vi "User_Metadata.vi"() -> ()   [LabVIEW 2010]
uses:
  ADAM Controls/Channel_names.ctl
  ADAM Controls/Module_type_ADAM.ctl
  ADAM Controls/Channel_State.ctl
  ADAM Controls/Calib_type_ADAM.ctl
  Anemometry/Anemometry Sub Vis/Controls/Preference_Mode.ctl
  ADAM Controls/Update_scan_value.ctl
  Anemometry/Anemometry Sub Vis/Globals/Preference_global.vi
  Anemometry/Anemometry Sub Vis/Globals/Constants_global.vi
  Anemometry/Anemometry Sub Vis/Globals/Meas_global.vi
  Anemometry/Anemometry Sub Vis/Globals/Trav_pos_global.vi
panel:
  in  "Edit Preference Panel":bool
  out "Rig Name":string="EnFlo Tunnel"
  in  "Edit Email Addresses":bool
  out "Email Addresses":string[](array[string])
  in  "Value 10":string
  in  "Value 9":string
  in  "Value 8":string
  in  "Value 7":string
  in  "Value 6":string
  in  "Menu 10":u16(ring) items=["Edit Strings", "20mm Cubes"]
  out "Channel Name 10":string
  in  "Menu 9":u16(ring) items=["Edit Strings", "None", "Ramp 29 x 390mm", "Ramp 9 x 175mm", "Rounded nose 18.2 x 55mm", "Rounded nose 9 x 150mm"]
  out "Channel Name 9":string
  in  "Menu 8":u16(ring) items=["Edit Strings", "20mm Cubes"]
  out "Channel Name 8":string
  in  "Menu 7":u16(ring) items=["Edit Strings", "0", "115", "65"]
  out "Channel Name 7":string
  in  "Menu 6":u16(ring) items=["Edit Strings", "0", "1", "16"]
  out "Channel Name 6":string
  out "Clear remaining channels":bool
  in  "Value 5":string
  in  "Menu 5":u16(ring) items=["Edit Strings", "0", "25", "6.25"]
  out "Channel Name 5":string
  in  "Value 4":string
  in  "Menu 4":u16(ring) items=["Edit Strings", "20 x 20mm", "40 x 40mm", "80 x 80mm", "None"]
  out "Channel Name 4":string
  in  "Value 3":string
  in  "Menu 3":u16(ring) items=["Edit Strings", "0", "10", "20", "Normal distribution with average = 10mm"]
  out "Channel Name 3":string
  in  "Value 2":string
  in  "Menu 2":u16(ring) items=["Edit Strings", "None", "Random blocks", "Uniform cube"]
  out "Channel Name 2":string
  in  "Modify User Channels":bool
  out "Channel No":i32
  out "First Loop":bool
  out "Index":i32
  in  "Value 1":string
  in  "Menu 1":u16(ring) items=["Edit Strings", "Aligned", "None", "Staggered"]
  out "Channel Name 1":string
  in  "stop":bool
  in  "OK":bool
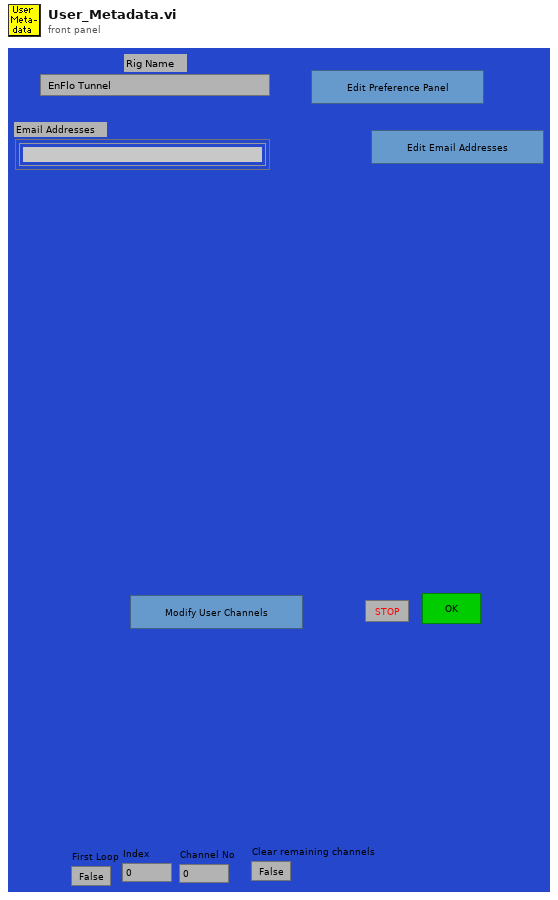
[diagram p1: front panel]
types:
  T1 = typedef "Channel_names.ctl" = enum16{"Active Only", "Active + Off", "All Channels"}
  T2 = typedef "Calib_type_ADAM.ctl" = enum16{"Raw", "Bx + A", "Cx^2 + Bx + A", "Dx^3 + Cx^2 + Bx + A", "In Band", "Hi-Tec Q", "Hi-Tec M_dot", "Text"}
  T3 = typedef "Preference_Mode.ctl" = enum16{"Load Preferences from file", "Save Preferences to file", "Load, Edit then Save"}
  T4 = typedef "Channel_State.ctl" = enum16{"On", "Off", "Always On", "Always Off"}
  T5 = typedef "Module_type_ADAM.ctl" = enum16{"4011", "4012", "4013", "4014", "4016", "4017", "4018", "4021", "4050", "4052", "4053", "4060", "4080", "5000", "5017", "5018", "5024", "5051", "5056", "5060", "6060", "Tracker", "WEST", "GILL", "JEM", "VICI", "Vaisala", "DRUCK", "Run VI Named:", "IR2100", "PPT", "Comparator", "VIRTUAL", "Hold Value", "Read A", "Read Ch", "Coded", "Client Info", "Web Client", "X10", "Test"}
  T6 = typedef "Ch_description_ADAM.ctl" = cluster{"Ch Name":string, "Type":T5, "Function":T7, "Ch State":T4, "Calibration type":T2, "A":dbl, "B":dbl, "C":dbl, "D":dbl, "Comments":string, "Address":T8, "String":string, "Duty":u16}
  T7 = typedef "Function_ADAM.ctl" = enum16{"Analogue Input", "Digital Input", "Event counter", "Event rate", "Analogue Output", "Digital Output", "Relay Output"}
  T8 = typedef "Address.ctl" = cluster{"Main":i32, "Ch.":i32, "Sub":i32, "Port Name":string}
  T9 = typedef "Update_scan_value.ctl" = cluster{"Channel Name":string, "New Value":dbl}
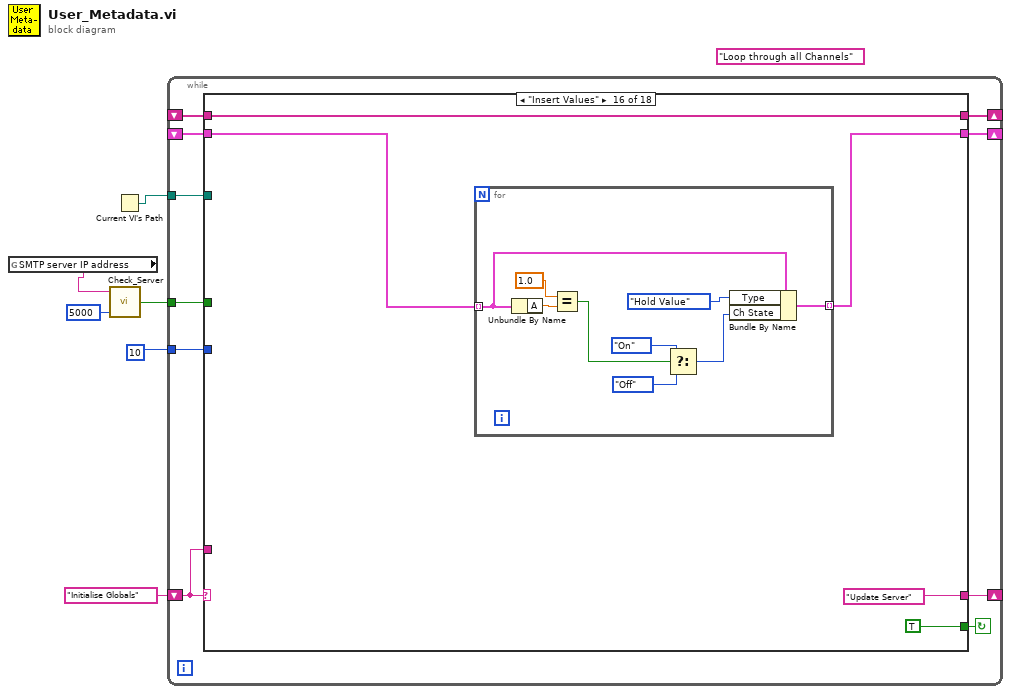
[diagram p0: block diagram]
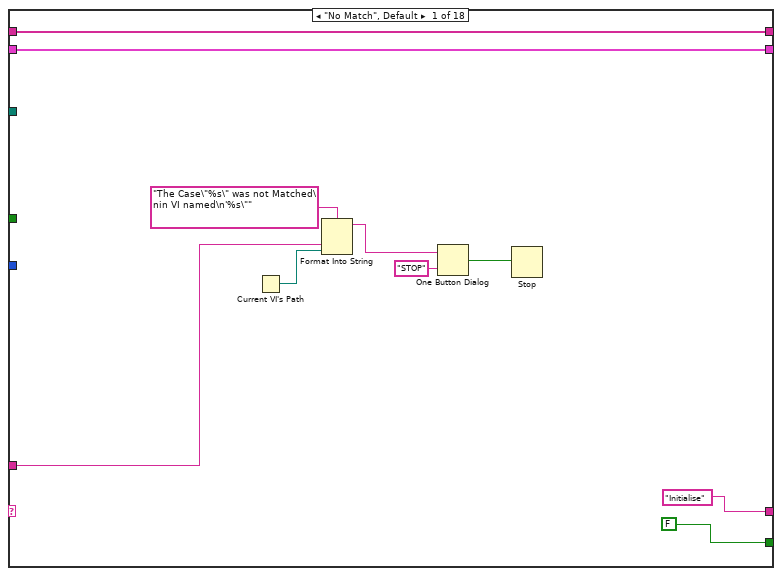
[diagram p2: hidden frame]
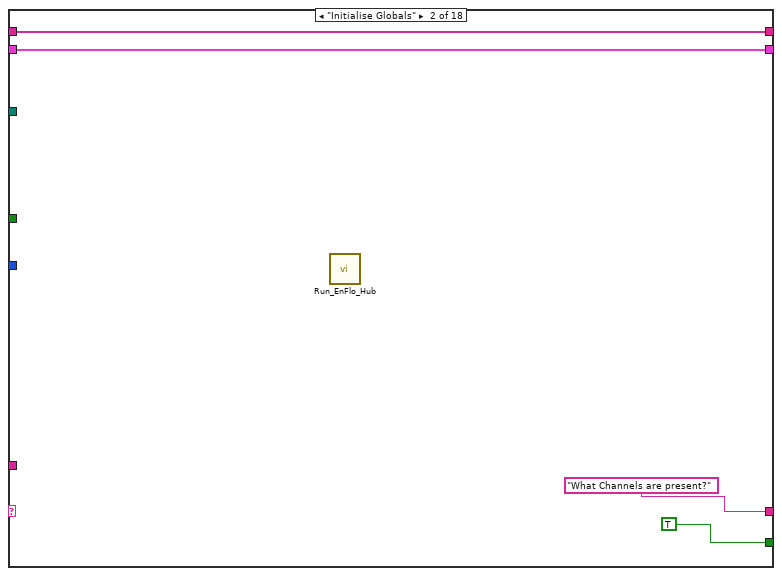
[diagram p3: hidden frame]
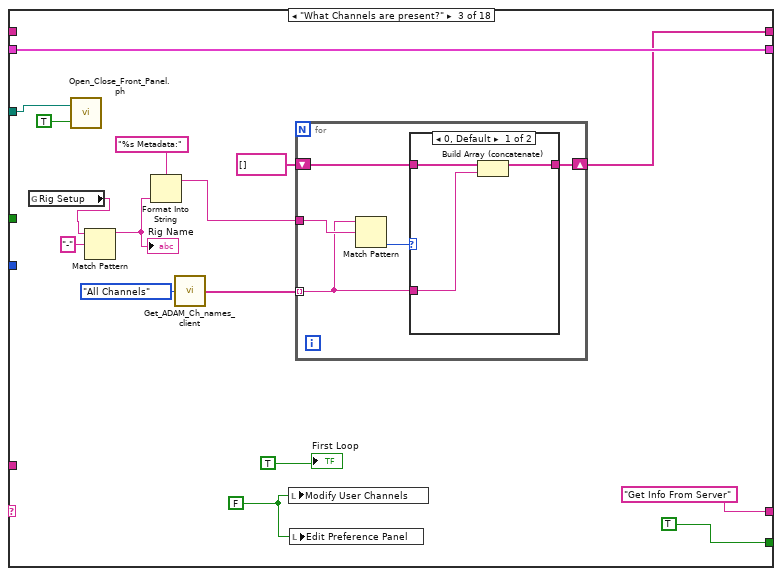
[diagram p4: hidden frame]
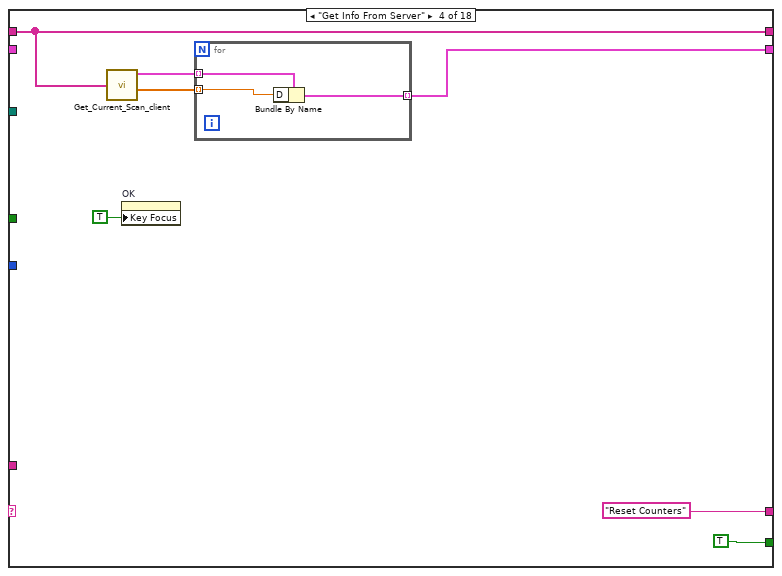
[diagram p6: hidden frame]
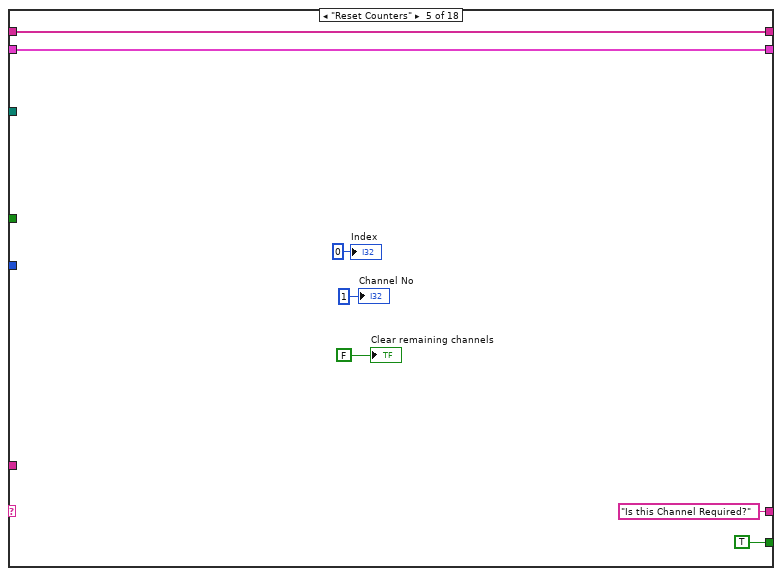
[diagram p7: hidden frame]
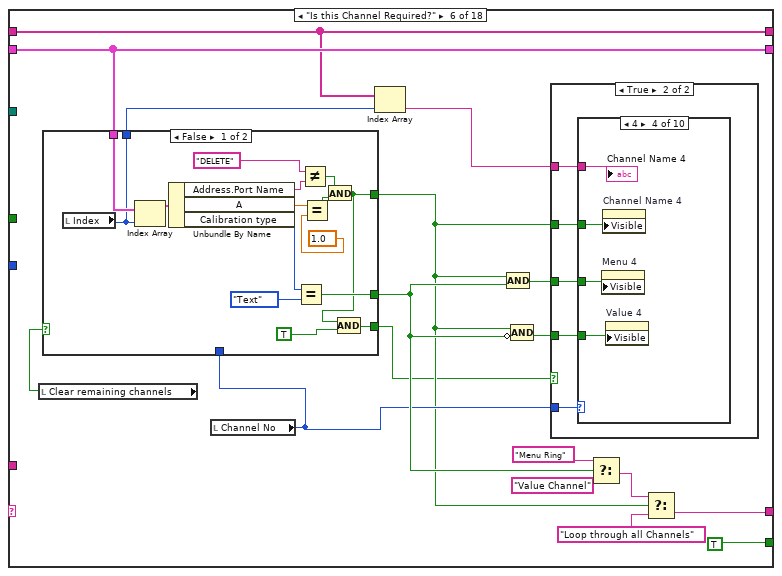
[diagram p8: hidden frame]
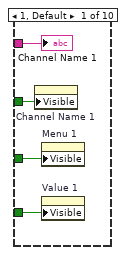
[diagram p10: hidden frame]
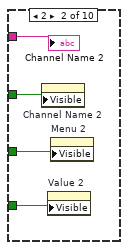
[diagram p11: hidden frame]
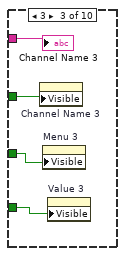
[diagram p12: hidden frame]
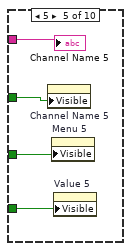
[diagram p13: hidden frame]
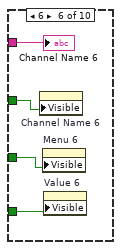
[diagram p14: hidden frame]
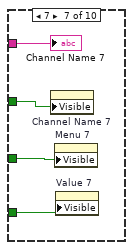
[diagram p15: hidden frame]
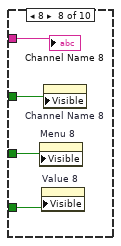
[diagram p16: hidden frame]
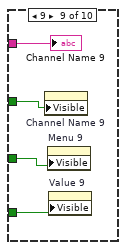
[diagram p17: hidden frame]
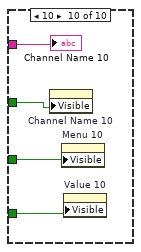
[diagram p18: hidden frame]
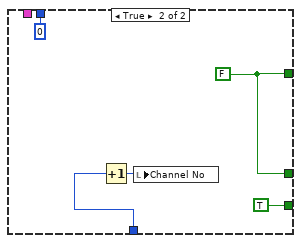
[diagram p19: hidden frame]
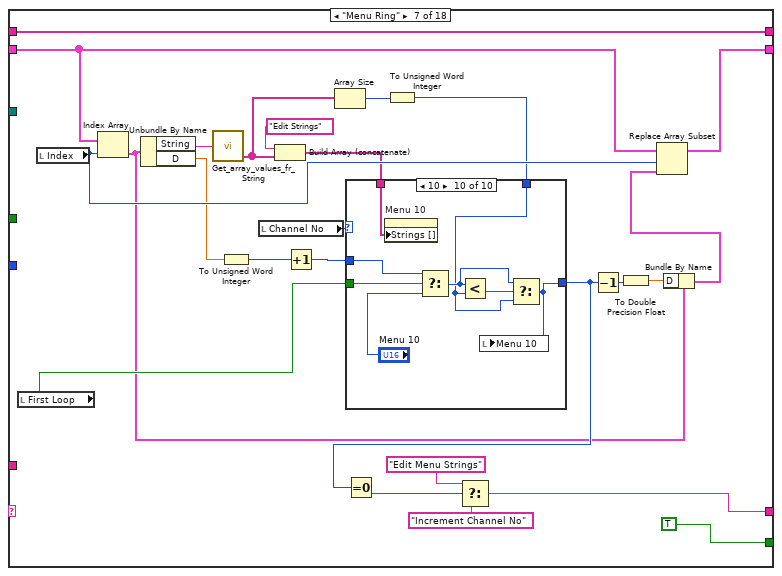
[diagram p20: hidden frame]
diagram:
  (unwired) "Loop through all Channels"
  n1 = global read "Preference_global.vi" "SMTP server IP address"() -> (w2:string)
  n2 = call "Check_Server.vi"("timeout ms (60000)"=5000, "address"=w2) -> ("OK"=w1:bool)  [unwired: 3 out]
  n3 = Current VI's Path() -> (path=w4:path)
  n4 = while {
    tunnel: 10 -> [w9]
    shift-left: _ -> [w12]
    shift-right: [w11] -> _
    shift-left: _ -> [w13]
    shift-right: [w14] -> _
    shift-left: "Initialise Globals" -> [w15]
    shift-right: [w10] -> _
    tunnel: w4 -> [w8]
    tunnel: w1 -> [w7]
    stop <- w16 continue-if-true
    n5 = case shown="\"Insert Values\"" w15 {
      tunnel: [FALSE TRUE TRUE TRUE TRUE ("T button?") TRUE TRUE TRUE TRUE TRUE TRUE TRUE TRUE TRUE ("T button?") TRUE ("T button?") TRUE ("T button?") TRUE ("T button?") FALSE ("T button?")] -> w16
      tunnel: ["Initialise" "What Channels are present?" "Get Info From Server" "Reset Counters" "Is this Channel Required?" w84 w166 "Increment Channel No" "Increment Channel No" "Loop through all Channels" w347 "What Channels are present?" "Reset Counters" w396 "Insert Values" "Update Server" w439 "End"] -> w10
      tunnel: w15 -> [w21 _ _ _ _ _ _ _ _ _ _ _ _ _ _ _ _ _]
      tunnel: [w18 w28 w44 w57 w69 w88 w158 w269 w287 w345 w358 w379 w384 w406 w419 w427 w440 w487] -> w14
      tunnel: w13 -> [w18 w28 w44 _ w69 w88 w159 w268 w288 w345 w358 w379 w385 w406 w419 w425 w440 w487]
      tunnel: w12 -> [w17 w27 _ w60 w70 w78 w178 w273 w298 w344 w363 w380 _ w399 w417 w426 w441 w488]
      tunnel: [w17 w27 w40 w60 w70 w78 w178 w273 w298 w344 w363 w380 w383 w399 w417 w426 w441 w488] -> w11
      tunnel: w9 -> [_ _ _ _ _ _ _ _ _ _ w353 _ _ _ _ _ _ _]
      tunnel: w8 -> [_ _ w35 _ _ _ _ _ _ _ _ _ _ _ _ _ _ w485]
      tunnel: w7 -> [_ _ _ _ _ _ _ _ _ _ _ _ _ _ w412 _ _ _]
      frame "No Match", Default {
        n6 = Current VI's Path() -> (path=w20:path)
        n7 = Format Into String(format string="The Case\"%s\" was not Matched\nin VI named\n'%s\"" ("Format String"), w21, w20) -> (resulting string=w24:string)  [unwired: 2 in, 1 out]
        n8 = One Button Dialog(message=w24, button name ("OK")="STOP") -> (true=w22:bool)
        n9 = Stop(stop? (T)=w22) -> ()
      }
      frame "Initialise Globals" {
        n10 = call "Run_EnFlo_Hub.vi"() -> ()  [unwired: 8 out]
      }
      frame "What Channels are present?" {
        w34 = FALSE ("Add a New Channel")
        n11 = global read "Preference_global.vi" "Rig Setup"() -> (w32:string)
        n12 = call "Open_Close_Front_Panel.ph.vi"("Front Panel Window:Open"=TRUE, "VI path"=w35) -> ()  [unwired: 2 out]
        n13 = Match Pattern(string=w32, regular expression="-") -> (before substring=w31:string)  [unwired: 4 out]
        "Rig Name" <- w31
        n14 = Format Into String(format string="%s Metadata:" ("Format String"), w31) -> (resulting string=w37:string)  [unwired: 2 in, 1 out]
        n15 = call "Get_ADAM_Ch_names_client.vi"("Channel names set"=Channel_names."All Channels") -> ("Ch names"=w42:string[])
        n16 = local write "Modify User Channels"(w34) -> ()
        n17 = local write "Edit Preference Panel"(w34) -> ()
        n18 = for {
          tunnel: w37 -> [w51]
          tunnel: w42 -> [w49] mode=indexing
          shift-right: [w47] -> w40
          shift-left: string[] [] -> [w48]
          n19 = Match Pattern(string=w49, regular expression=w51) -> (offset past match=w50:i32)  [unwired: 4 out]
          n20 = case shown="0, Default" w50 {
            tunnel: w49 -> [w54 _]
            tunnel: w48 -> [w53 w55]
            tunnel: [w52 w55] -> w47
            frame 0, Default {
              n21 = Build Array (concatenate)(w53, w54) -> (w52:string[])
            }
            frame -1 {
            }
          }
        }
        "First Loop" <- TRUE ("First Loop")
      }
      frame "Get Info From Server" {
        n22 = call "Get_Current_Scan_client.vi"("ADAM Ch Names"=w60) -> ("Ch Description Array"=w59:T6[], "Numerical Values"=w58:dbl[])  [unwired: 2 out]
        n23 = property on="OK" class="Bool"("Key Focus"=TRUE) -> ()  [unwired: 2 in, 2 out]
        n24 = for {
          tunnel: w59 -> [w65] mode=indexing
          tunnel: w58 -> [w64] mode=indexing
          tunnel: [w63] -> w57 mode=indexing
          n25 = Bundle By Name(cluster=w65, "D"=w64) -> (w63:T6)
        }
      }
      frame "Reset Counters" {
        "Index" <- 0 ("Index")
        "Channel No" <- 1 ("Channel No")
        "Clear remaining channels" <- FALSE ("Clear remaining channels")
      }
      frame "Is this Channel Required?" {
        n26 = local read "Clear remaining channels"() -> (w76:bool)
        n27 = local read "Channel No"() -> (w75:i32)
        n28 = case shown="False" w76 {
          tunnel: w88 -> [w149 _]
          tunnel: [w135 w154] -> w74
          tunnel: [w145 w154] -> w83
          tunnel: [w144 0 ("Index")] -> w79
          tunnel: w75 -> [_ w151]
          tunnel: [w142 TRUE] -> w73
          frame False {
            n29 = local read "Index"() -> (w144:i32)
            n30 = Index Array(array=w149, index=w144) -> (element=w148:T6)
            n31 = Unbundle By Name(w148) -> ("Address.Port Name"=w139:string, "A"=w141:dbl, "Calibration type"=w146:T2)
            n32 = Equal?(x=w146, y=Calib_type_ADAM."Text" ("Calibration Type")) -> (x = y?=w145:bool)
            n33 = Not Equal?(x="DELETE", y=w139) -> (x != y?=w136:bool)
            n34 = Equal?(x=w141, y=1.0 ("x")) -> (x = y?=w137:bool)
            n35 = And(x=w136, y=w137) -> (x .and. y?=w135:bool)
            n36 = Compound Arithmetic op=AND(w135, TRUE ("Input")) -> (w142:bool)
          }
          frame True {
            w154 = FALSE
            n37 = Increment(x=w151) -> (x+1=w152:i32)
            n38 = local write "Channel No"(w152) -> ()
          }
        }
        n39 = Index Array(array=w78, index=w79) -> (element=w77:string)
        n40 = Compound Arithmetic op=AND(w74, w83) -> (w86:bool)
        n41 = Compound Arithmetic op=AND(w74, invert w83) -> (w87:bool)
        n42 = case shown="True" w73 {
          tunnel: w87 -> [_ w94]
          tunnel: w86 -> [_ w93]
          tunnel: w74 -> [_ w92]
          tunnel: w77 -> [_ w91]
          tunnel: w75 -> [_ w90]
          frame False {
          }
          frame True {
            n43 = case shown="4" w90 {
              tunnel: w92 -> [w96 w100 w104 w108 w112 w117 w121 w125 w129 w133]
              tunnel: w94 -> [w98 w102 w106 w110 w114 w115 w119 w123 w127 w131]
              tunnel: w93 -> [w97 w101 w105 w109 w113 w116 w120 w124 w128 w134]
              tunnel: w91 -> [w95 w99 w103 w107 w111 w118 w122 w126 w130 w132]
              frame 1, Default {
                n44 = property on="Channel Name 1" class="Str"("Visible"=w96) -> ()  [unwired: 2 in, 2 out]
                n45 = property on="Menu 1" class="Ring (strict)"("Visible"=w97) -> ()  [unwired: 2 in, 2 out]
                n46 = property on="Value 1" class="Str"("Visible"=w98) -> ()  [unwired: 2 in, 2 out]
                "Channel Name 1" <- w95
              }
              frame 2 {
                n47 = property on="Channel Name 2" class="Str"("Visible"=w100) -> ()  [unwired: 2 in, 2 out]
                n48 = property on="Value 2" class="Str"("Visible"=w102) -> ()  [unwired: 2 in, 2 out]
                n49 = property on="Menu 2" class="Ring (strict)"("Visible"=w101) -> ()  [unwired: 2 in, 2 out]
                "Channel Name 2" <- w99
              }
              frame 3 {
                n50 = property on="Channel Name 3" class="Str"("Visible"=w104) -> ()  [unwired: 2 in, 2 out]
                n51 = property on="Menu 3" class="Ring (strict)"("Visible"=w105) -> ()  [unwired: 2 in, 2 out]
                n52 = property on="Value 3" class="Str"("Visible"=w106) -> ()  [unwired: 2 in, 2 out]
                "Channel Name 3" <- w103
              }
              frame 4 {
                n53 = property on="Menu 4" class="Ring (strict)"("Visible"=w109) -> ()  [unwired: 2 in, 2 out]
                n54 = property on="Channel Name 4" class="Str"("Visible"=w108) -> ()  [unwired: 2 in, 2 out]
                n55 = property on="Value 4" class="Str"("Visible"=w110) -> ()  [unwired: 2 in, 2 out]
                "Channel Name 4" <- w107
              }
              frame 5 {
                n56 = property on="Channel Name 5" class="Str"("Visible"=w112) -> ()  [unwired: 2 in, 2 out]
                n57 = property on="Menu 5" class="Ring (strict)"("Visible"=w113) -> ()  [unwired: 2 in, 2 out]
                n58 = property on="Value 5" class="Str"("Visible"=w114) -> ()  [unwired: 2 in, 2 out]
                "Channel Name 5" <- w111
              }
              frame 6 {
                n59 = property on="Channel Name 6" class="Str"("Visible"=w117) -> ()  [unwired: 2 in, 2 out]
                n60 = property on="Menu 6" class="Ring (strict)"("Visible"=w116) -> ()  [unwired: 2 in, 2 out]
                n61 = property on="Value 6" class="Str"("Visible"=w115) -> ()  [unwired: 2 in, 2 out]
                "Channel Name 6" <- w118
              }
              frame 7 {
                n62 = property on="Channel Name 7" class="Str"("Visible"=w121) -> ()  [unwired: 2 in, 2 out]
                n63 = property on="Menu 7" class="Ring (strict)"("Visible"=w120) -> ()  [unwired: 2 in, 2 out]
                n64 = property on="Value 7" class="Str"("Visible"=w119) -> ()  [unwired: 2 in, 2 out]
                "Channel Name 7" <- w122
              }
              frame 8 {
                n65 = property on="Menu 8" class="Ring (strict)"("Visible"=w124) -> ()  [unwired: 2 in, 2 out]
                n66 = property on="Value 8" class="Str"("Visible"=w123) -> ()  [unwired: 2 in, 2 out]
                n67 = property on="Channel Name 8" class="Str"("Visible"=w125) -> ()  [unwired: 2 in, 2 out]
                "Channel Name 8" <- w126
              }
              frame 9 {
                n68 = property on="Channel Name 9" class="Str"("Visible"=w129) -> ()  [unwired: 2 in, 2 out]
                n69 = property on="Menu 9" class="Ring (strict)"("Visible"=w128) -> ()  [unwired: 2 in, 2 out]
                n70 = property on="Value 9" class="Str"("Visible"=w127) -> ()  [unwired: 2 in, 2 out]
                "Channel Name 9" <- w130
              }
              frame 10 {
                n71 = property on="Channel Name 10" class="Str"("Visible"=w133) -> ()  [unwired: 2 in, 2 out]
                n72 = property on="Menu 10" class="Ring (strict)"("Visible"=w134) -> ()  [unwired: 2 in, 2 out]
                n73 = property on="Value 10" class="Str"("Visible"=w131) -> ()  [unwired: 2 in, 2 out]
                "Channel Name 10" <- w132
              }
            }
          }
        }
        n74 = Select(t="Menu Ring", s=w83, f="Value Channel") -> (s? t:f=w81:string)
        n75 = Select(t=w81, s=w74, f="Loop through all Channels") -> (s? t:f=w84:string)
      }
      frame "Menu Ring" {
        n76 = local read "First Loop"() -> (w176:bool)
        n77 = local read "Index"() -> (w171:i32)
        n78 = Index Array(array=w159, index=w171) -> (element=w156:T6)
        n79 = Unbundle By Name(w156) -> ("String"=w177:string, "D"=w160:dbl)
        n80 = call "Get_array_values_fr_String.vi"("String Value"=w177) -> ("String array"=w164:string[])  [unwired: 1 out]
        n81 = To Unsigned Word Integer(number=w160) -> (unsigned 16bit integer=w175:u16)
        n82 = local read "Channel No"() -> (w170:i32)
        n83 = Build Array (concatenate)("Edit Strings", w164) -> (w165:string[])
        n84 = Increment(x=w175) -> (x+1=w173:u16)
        n85 = Array Size(array=w164) -> (size(s)=w163:i32)
        n86 = To Unsigned Word Integer(number=w163) -> (unsigned 16bit integer=w162:u16)
        n87 = case shown="10" w170 {
          tunnel: w176 -> [w186 w195 w203 w211 w219 w227 w235 w243 w251 w259]
          tunnel: w173 -> [w185 w194 w202 w210 w218 w226 w234 w242 w250 w258]
          tunnel: [w180 w190 w198 w206 w214 w222 w230 w238 w246 w254] -> w172
          tunnel: w165 -> [w184 w188 w197 w205 w213 w220 w229 w237 w245 w253]
          tunnel: w162 -> [w181 w191 w199 w207 w215 w223 w231 w239 w247 w255]
          frame 1, Default {
            n88 = property on="Menu 1" class="Ring (strict)"("Strings []"=w184) -> ()  [unwired: 2 in, 2 out]
            n89 = Select(t=w185, s=w186, f="Menu 1") -> (s? t:f=w182:u16)
            n90 = Less?(x=w182, y=w181) -> (x < y?=w183:bool)
            n91 = Select(t=w182, s=w183, f=w181) -> (s? t:f=w180:u16)
            n92 = local write "Menu 1"(w180) -> ()
          }
          frame 2 {
            n93 = property on="Menu 2" class="Ring (strict)"("Strings []"=w188) -> ()  [unwired: 2 in, 2 out]
            n94 = Select(t=w194, s=w195, f="Menu 2") -> (s? t:f=w192:u16)
            n95 = Less?(x=w192, y=w191) -> (x < y?=w193:bool)
            n96 = Select(t=w192, s=w193, f=w191) -> (s? t:f=w190:u16)
            n97 = local write "Menu 2"(w190) -> ()
          }
          frame 3 {
            n98 = property on="Menu 3" class="Ring (strict)"("Strings []"=w197) -> ()  [unwired: 2 in, 2 out]
            n99 = Select(t=w202, s=w203, f="Menu 3") -> (s? t:f=w200:u16)
            n100 = Less?(x=w200, y=w199) -> (x < y?=w201:bool)
            n101 = Select(t=w200, s=w201, f=w199) -> (s? t:f=w198:u16)
            n102 = local write "Menu 3"(w198) -> ()
          }
          frame 4 {
            n103 = property on="Menu 4" class="Ring (strict)"("Strings []"=w205) -> ()  [unwired: 2 in, 2 out]
            n104 = Select(t=w210, s=w211, f="Menu 4") -> (s? t:f=w208:u16)
            n105 = Less?(x=w208, y=w207) -> (x < y?=w209:bool)
            n106 = Select(t=w208, s=w209, f=w207) -> (s? t:f=w206:u16)
            n107 = local write "Menu 4"(w206) -> ()
          }
          frame 5 {
            n108 = property on="Menu 5" class="Ring (strict)"("Strings []"=w213) -> ()  [unwired: 2 in, 2 out]
            n109 = Select(t=w218, s=w219, f="Menu 5") -> (s? t:f=w216:u16)
            n110 = Less?(x=w216, y=w215) -> (x < y?=w217:bool)
            n111 = Select(t=w216, s=w217, f=w215) -> (s? t:f=w214:u16)
            n112 = local write "Menu 5"(w214) -> ()
          }
          frame 6 {
            n113 = property on="Menu 6" class="Ring (strict)"("Strings []"=w220) -> ()  [unwired: 2 in, 2 out]
            n114 = Select(t=w226, s=w227, f="Menu 6") -> (s? t:f=w224:u16)
            n115 = Less?(x=w224, y=w223) -> (x < y?=w225:bool)
            n116 = Select(t=w224, s=w225, f=w223) -> (s? t:f=w222:u16)
            n117 = local write "Menu 6"(w222) -> ()
          }
          frame 7 {
            n118 = property on="Menu 7" class="Ring (strict)"("Strings []"=w229) -> ()  [unwired: 2 in, 2 out]
            n119 = Select(t=w234, s=w235, f="Menu 7") -> (s? t:f=w232:u16)
            n120 = Less?(x=w232, y=w231) -> (x < y?=w233:bool)
            n121 = Select(t=w232, s=w233, f=w231) -> (s? t:f=w230:u16)
            n122 = local write "Menu 7"(w230) -> ()
          }
          frame 8 {
            n123 = property on="Menu 8" class="Ring (strict)"("Strings []"=w237) -> ()  [unwired: 2 in, 2 out]
            n124 = Select(t=w242, s=w243, f="Menu 8") -> (s? t:f=w240:u16)
            n125 = Less?(x=w240, y=w239) -> (x < y?=w241:bool)
            n126 = Select(t=w240, s=w241, f=w239) -> (s? t:f=w238:u16)
            n127 = local write "Menu 8"(w238) -> ()
          }
          frame 9 {
            n128 = property on="Menu 9" class="Ring (strict)"("Strings []"=w245) -> ()  [unwired: 2 in, 2 out]
            n129 = Select(t=w250, s=w251, f="Menu 9") -> (s? t:f=w248:u16)
            n130 = Less?(x=w248, y=w247) -> (x < y?=w249:bool)
            n131 = Select(t=w248, s=w249, f=w247) -> (s? t:f=w246:u16)
            n132 = local write "Menu 9"(w246) -> ()
          }
          frame 10 {
            n133 = property on="Menu 10" class="Ring (strict)"("Strings []"=w253) -> ()  [unwired: 2 in, 2 out]
            n134 = Select(t=w258, s=w259, f="Menu 10") -> (s? t:f=w256:u16)
            n135 = Less?(x=w256, y=w255) -> (x < y?=w257:bool)
            n136 = Select(t=w256, s=w257, f=w255) -> (s? t:f=w254:u16)
            n137 = local write "Menu 10"(w254) -> ()
          }
        }
        n138 = Equal To 0?(x=w172) -> (x = 0?=w169:bool)
        n139 = Select(t="Edit Menu Strings", s=w169, f="Increment Channel No") -> (s? t:f=w166:string)
        n140 = Decrement(x=w172) -> (x-1=w161:u16)
        n141 = To Double Precision Float(number=w161) -> (double precision float=w157:dbl)
        n142 = Bundle By Name(cluster=w156, "D"=w157) -> (w155:T6)
        n143 = Replace Array Subset(array=w159, new element=w155, index=w171) -> (w158:T6[])
      }
      frame "Edit Menu Strings" {
        n144 = local read "Index"() -> (w263:i32)
        n145 = Index Array(array=w268, index=w263) -> (element=w272:T6)
        n146 = Unbundle By Name(w272) -> ("String"=w274:string, "Ch Name"=w262:string)
        n147 = call "Get_array_values_fr_String.vi"("String Value"=w274) -> ("String array"=w267:string[])  [unwired: 1 out]
        n148 = call "Edit_String_Options_list.vi"("Channel Name"=w262, "String array"=w267) -> ("New Selection Index"=w260:i32, "String array Out"=w266:string[])
        n149 = call "Put_Array_into_String.vi"("String array"=w266) -> ("String Value"=w271:string)
        n150 = local read "Channel No"() -> (w265:i32)
        n151 = Increment(x=w260) -> (x+1=w264:i32)
        n152 = Bundle By Name(cluster=w272, "String"=w271, "D"=w260) -> (w270:T6)
        n153 = To Unsigned Word Integer(number=w264) -> (unsigned 16bit integer=w261:u16)
        n154 = case shown="5" w265 {
          tunnel: w261 -> [w277 w278 w279 w280 w281 w282 w283 w284 w285 w286]
          frame 1, Default {
            n155 = local write "Menu 1"(w277) -> ()
          }
          frame 2 {
            n156 = local write "Menu 2"(w278) -> ()
          }
          frame 3 {
            n157 = local write "Menu 3"(w279) -> ()
          }
          frame 4 {
            n158 = local write "Menu 4"(w280) -> ()
          }
          frame 5 {
            n159 = local write "Menu 5"(w281) -> ()
          }
          frame 6 {
            n160 = local write "Menu 6"(w282) -> ()
          }
          frame 7 {
            n161 = local write "Menu 7"(w283) -> ()
          }
          frame 8 {
            n162 = local write "Menu 8"(w284) -> ()
          }
          frame 9 {
            n163 = local write "Menu 9"(w285) -> ()
          }
          frame 10 {
            n164 = local write "Menu 10"(w286) -> ()
          }
        }
        n165 = Replace Array Subset(array=w268, new element=w270, index=w263) -> (w269:T6[])
      }
      frame "Value Channel" {
        n166 = local read "Index"() -> (w297:i32)
        n167 = local read "First Loop"() -> (w295:bool)
        n168 = Index Array(array=w288, index=w297) -> (element=w289:T6)
        n169 = local read "Channel No"() -> (w296:i32)
        n170 = Unbundle By Name(w289) -> ("D"=w291:dbl)
        n171 = call "Number_2_string.vi"("number"=w291) -> ("String"=w294:string)  [unwired: 1 in]
        n172 = case shown="1, Default" w296 {
          tunnel: w295 -> [w304 w308 w312 w316 w320 w324 w328 w332 w336 w340]
          tunnel: w294 -> [w303 w307 w311 w315 w319 w323 w327 w331 w335 w339]
          tunnel: [w301 w306 w310 w314 w318 w322 w326 w330 w334 w338] -> w293
          frame 1, Default {
            n173 = Select(t=w303, s=w304, f="Value 1") -> (s? t:f=w301:string)
            n174 = local write "Value 1"(w301) -> ()
          }
          frame 2 {
            n175 = Select(t=w307, s=w308, f="Value 2") -> (s? t:f=w306:string)
            n176 = local write "Value 2"(w306) -> ()
          }
          frame 3 {
            n177 = Select(t=w311, s=w312, f="Value 3") -> (s? t:f=w310:string)
            n178 = local write "Value 3"(w310) -> ()
          }
          frame 4 {
            n179 = Select(t=w315, s=w316, f="Value 4") -> (s? t:f=w314:string)
            n180 = local write "Value 4"(w314) -> ()
          }
          frame 5 {
            n181 = Select(t=w319, s=w320, f="Value 5") -> (s? t:f=w318:string)
            n182 = local write "Value 5"(w318) -> ()
          }
          frame 6 {
            n183 = Select(t=w323, s=w324, f="Value 6") -> (s? t:f=w322:string)
            n184 = local write "Value 6"(w322) -> ()
          }
          frame 7 {
            n185 = Select(t=w327, s=w328, f="Value 7") -> (s? t:f=w326:string)
            n186 = local write "Value 7"(w326) -> ()
          }
          frame 8 {
            n187 = Select(t=w331, s=w332, f="Value 8") -> (s? t:f=w330:string)
            n188 = local write "Value 8"(w330) -> ()
          }
          frame 9 {
            n189 = Select(t=w335, s=w336, f="Value 9") -> (s? t:f=w334:string)
            n190 = local write "Value 9"(w334) -> ()
          }
          frame 10 {
            n191 = Select(t=w339, s=w340, f="Value 10") -> (s? t:f=w338:string)
            n192 = local write "Value 10"(w338) -> ()
          }
        }
        n193 = Fract/Exp String To Number(string=w293) -> (number=w292:dbl)  [unwired: 4 out]
        n194 = Bundle By Name(cluster=w289, "D"=w292) -> (w290:T6)
        n195 = Replace Array Subset(array=w288, new element=w290, index=w297) -> (w287:T6[])
      }
      frame "Increment Channel No" {
        n196 = local read "Channel No"() -> (w343:i32)
        n197 = Increment(x=w343) -> (x+1=w342:i32)
        n198 = local write "Channel No"(w342) -> ()
      }
      frame "Loop through all Channels" {
        n199 = local read "Index"() -> (w362:i32)
        n200 = Array Size(array=w358) -> (size(s)=w357:i32)
        n201 = local read "Channel No"() -> (w348:i32)
        n202 = Increment(x=w362) -> (x+1=w361:i32)
        n203 = Less?(x=w361, y=w357) -> (x < y?=w351:bool)
        n204 = local write "Index"(w361) -> ()
        n205 = Less Or Equal?(x=w348, y=w353) -> (x <= y?=w350:bool)
        n206 = Or(x=w351, y=w350) -> (x .or. y?=w352:bool)
        n207 = Compound Arithmetic op=AND(invert w351, w350) -> (w349:bool)
        n208 = case shown="False" w349 {
          frame False {
          }
          frame True {
            n209 = local write "Clear remaining channels"(TRUE ("Clear remaining channels")) -> ()
          }
        }
        n210 = Select(t="Is this Channel Required?", s=w352, f="Is User Ready Yet?") -> (s? t:f=w354:string)
        n211 = Select(t="Edit User Channels", s="Modify User Channels", f=w354) -> (s? t:f=w347:string)
      }
      frame "Edit Preference Panel" {
        n212 = global read "Constants_global.vi" "EnFlo SW Folder"() -> (w367:path)
        n213 = Build Path(base path=w367, name or relative path=path "Anemometry/Utilities/Preference_Panel.vi") -> (appended path=w370:path)
        n214 = Open VI Reference(type specifier VI Refnum (for type only)=refnum<vi> refnum, vi path=w370) -> (vi reference=w377:refnum<vi>, error out=w376:errorcluster)  [unwired: 1 in, 3 out]
        n215 = property class="VI Interface Type 0"(reference=w377, error in=w376, "Front Panel Window:Open"=TRUE) -> (reference out=w374:refnum<vi>, error out=w373:errorcluster)
        n216 = call-by-ref "?"(reference=w374, error in=w373, "Mode"=Preference_Mode."Load, Edit then Save") -> (reference out=w372:refnum<vi>, error out=w371:errorcluster)
        n217 = Close Reference(reference=w372, error in (no error)=w371) -> ()  [unwired: 1 out]
      }
      frame "Edit User Channels" {
        n218 = call "Modify_Metadata_Channels.vi"("Ch Description Array"=w385) -> ("Ch Description Array Out"=w384:T6[])  [unwired: 4 out]
        n219 = local write "First Loop"(TRUE ("First Loop")) -> ()
        n220 = for {
          tunnel: w384 -> [w390] mode=indexing
          tunnel: [w389] -> w383 mode=indexing
          n221 = Unbundle By Name(w390) -> ("Ch Name"=w389:string)
        }
        n222 = local write "Modify User Channels"(FALSE ("Add a New Channel")) -> ()
      }
      frame "Is User Ready Yet?" {
        w398 = FALSE ("First Loop")
        n223 = Or(x="stop", y="OK") -> (x .or. y?=w402:bool)
        n224 = case shown="False" "Edit Email Addresses" {
          frame False {
            n225 = global read "Meas_global.vi" "People to Email"() -> (w408:string[])
            "Email Addresses" <- w408
            n226 = Array Size(array=w408) -> (size(s)=w407:i32)
            n227 = property on="Email Addresses" class="Arr (strict)"("Number of Rows"=w407) -> ()  [unwired: 2 in, 2 out]
          }
          frame True {
            w409 = FALSE  # OK
            n228 = call "Get_users_email_addresses.vi"("OK"=w409) -> ()  [unwired: 5 out]
            n229 = local write "Edit Email Addresses"(FALSE ("Edit Email Addresses")) -> ()
          }
        }
        n230 = Current VI's Path() -> (path=w404:path)
        n231 = Or(x="stop", y="Edit Preference Panel") -> (x .or. y?=w392:bool)
        n232 = call "Close_Panel_and_Abort.vi"("Vi path"=w404, "stop"="stop") -> ()  [unwired: 1 out]
        n233 = Select(t="Valid User Name?", s=w402, f="Reset Counters") -> (s? t:f=w391:string)
        n234 = Select(t="Insert Values", s=w392, f=w391) -> (s? t:f=w396:string)
        n235 = local write "Clear remaining channels"(w398) -> ()
        n236 = local write "First Loop"(w398) -> ()
      }
      frame "Valid User Name?" {
        n237 = local read "Email Addresses"() -> (w416:string[])
        n238 = Array Size(array=w416) -> (size(s)=w415:i32)
        n239 = Equal To 0?(x=w415) -> (x = 0?=w413:bool)
        n240 = And(x=w412, y=w413) -> (x .and. y?=w414:bool)
        n241 = case shown="True" w414 {
          frame False {
          }
          frame True {
            n242 = Two Button Dialog(message="Are you sure you don't want to enter an email address?", 1:"Don't bother" ("F button name (\"Cancel\")"), 2:"Edit Email list" ("T button name (\"OK\")")) -> (T button?=w420:bool)
            n243 = case shown="True" w420 {
              frame False {
              }
              frame True {
                w424 = FALSE  # OK
                n244 = call "Get_users_email_addresses.vi"("OK"=w424) -> ()  [unwired: 5 out]
              }
            }
          }
        }
      }
      frame "Insert Values" {
        n245 = for {
          tunnel: w425 -> [w436] mode=indexing
          tunnel: [w430] -> w427 mode=indexing
          n246 = Unbundle By Name(w436) -> ("A"=w438:dbl)
          n247 = Equal?(x=1.0, y=w438) -> (x = y?=w434:bool)
          n248 = Select(t=Channel_State."On" ("Channel State"), s=w434, f=Channel_State."Off" ("Channel State")) -> (s? t:f=w431:T4)
          n249 = Bundle By Name(cluster=w436, "Type"=Module_type_ADAM."Hold Value" ("Module Type"), "Ch State"=w431) -> (w430:T6)
        }
      }
      frame "Update Server" {
        n250 = stacked-sequence {
          seq-local: [w445 _] -> [_ _]
          seq-local: [w443 _] -> [_ _]
          tunnel: w440 -> [w451 _]
          tunnel: [_ w480] -> w439
          frame #0 {
            w449 = T9 {"Channel Name"="", "New Value"=0.0} ("Update Scan Value Cluster")
            n251 = call "Update_Ch_Discription_client.vi"("Channels to update In"=w451) -> ()  [unwired: 1 out]
            n252 = Initialize Array(w449, 0 ("dimension size")) -> (w450:T9[])
            n253 = for {
              tunnel: w449 -> [w465]
              tunnel: w451 -> [w464] mode=indexing
              shift-right: [w457] -> w447
              shift-left: w450 -> [w458]
              shift-right: [w454] -> w445
              shift-left: i32[] [] -> [w455]
              shift-right: [w452] -> w443
              shift-left: dbl[] [] -> [w453]
              i -> [w456]
              n254 = Unbundle By Name(w464) -> ("Address.Port Name"=w461:string, "Ch Name"=w462:string, "D"=w463:dbl)
              n255 = Not Equal?(x="DELETE", y=w461) -> (x != y?=w459:bool)
              n256 = case shown="True" w459 {
                tunnel: w465 -> [_ w479]
                tunnel: w463 -> [_ w471]
                tunnel: w462 -> [_ w478]
                tunnel: w458 -> [w468 w477]
                tunnel: [w468 w476] -> w457
                tunnel: w456 -> [_ w474]
                tunnel: w455 -> [w467 w473]
                tunnel: [w467 w472] -> w454
                tunnel: w453 -> [w466 w470]
                tunnel: [w466 w469] -> w452
                frame False {
                }
                frame True {
                  n257 = Bundle By Name(cluster=w479, "Channel Name"=w478, "New Value"=w471) -> (w475:T9)
                  n258 = Build Array (concatenate)(w477, w475) -> (w476:T9[])
                  n259 = Build Array (concatenate)(w473, w474) -> (w472:i32[])
                  n260 = Build Array (concatenate)(w470, w471) -> (w469:dbl[])
                }
              }
            }
            n261 = call "Update_Current_Value_client.vi"("Update array in"=w447) -> ()  [unwired: 1 in]
          }
          frame #1 {
            n262 = local read "Edit Preference Panel"() -> (w483:bool)
            n263 = Select(t="Edit Preference Panel", s=w483, f="Close Panel") -> (s? t:f=w480:string)
          }
        }
      }
      frame "Close Panel" {
        n264 = call "Open_Close_Front_Panel.ph.vi"("Front Panel Window:Open"=FALSE, "VI path"=w485) -> ()  [unwired: 2 out]
        n265 = global write "Trav_pos_global.vi" "Show User Metadata on Launch?"(FALSE) -> ()
      }
    }
  }
